vi "TrajectoryGenerate_Make_Cubic_CtrlVect.vi"(8 "traj_config":T7={"MaxVelocity"=0.0, "Max Acceleration"=0.0, "StartVelocity"=0.0, "End Velocity"=0.0, "Reversed"=FALSE, "DiffDrKineConstntDefined"=FALSE, "CentAcellConstntDefined"=FALSE, "DiffDrVoltConstntDefined"=FALSE, "DIFF_DRIVE_KINE_CONSTRAINT"={"Max Speed (M/S)"=0.0, "DIFF_DRIVE_KINEMATICS"={"TrackWidth_Meters"=0.0}}, "CENTRIPETAL_ACCEL_CONSTRAINT"={"Max Cent Accel"=0.0}, "SwerveDrKineConstntDefined"=FALSE, "SWERVE_DRIVE_KINE_CONSTRAINT"={"Max Speed (M/S)"=0.0, "SwerveKinematics"={"NumModules"=0, "InverseKinematics"=[], "ForwardKinematics"=[], "Modules"=[], "PrevCoR"={"X"=0.0, "Y"=0.0}}}, "DIFF_DRIVE_VOLTAGE_CONSTRAINT"={"Max Voltage"=0.0, "DIFF_DRIVE_KINEMATICS"={"TrackWidth_Meters"=0.0}, "SIMPLE_MOTOR_FF"={"Ks"=0.0, "Kv"=0.0, "Ka"=0.0}}, "MECANUM_DRIVE_KINE_CONSTRAINT"={"Max Speed (M/S)"=0.0, "MECA_DRIVE_KINEMATICS"={"FrontLeft"={"X"=0.0, "Y"=0.0}, "FrontRight"={"X"=0.0, "Y"=0.0}, "RearLeft"={"X"=0.0, "Y"=0.0}, "RearRight"={"X"=0.0, "Y"=0.0}, "InverseKinematics"=[[0.0, 1.0, -1.0, 0.0], [0.0, 1.0, 1.0, 0.0], [0.0, 1.0, 1.0, 0.0], [0.0, 1.0, -1.0, 0.0]], "ForwardKinematics"=[[0.0, 1.0, -1.0, 0.0], [0.0, 1.0, 1.0, 0.0], [0.0, 1.0, 1.0, 0.0], [0.0, 1.0, -1.0, 0.0]], "PrevCoR"={"X"=0.0, "Y"=0.0}}}, "MecanumDrKineConstntDefined"=FALSE} {"MECANUM_DRIVE_KINE_CONSTRAINT"."MECA_DRIVE_KINEMATICS"."PrevCoR"."Y" format="%14.3f"; "MECANUM_DRIVE_KINE_CONSTRAINT"."MECA_DRIVE_KINEMATICS"."PrevCoR"."X" format="%14.3f"; "MECANUM_DRIVE_KINE_CONSTRAINT"."MECA_DRIVE_KINEMATICS"."RearRight"."Y" format="%14.3f"; "MECANUM_DRIVE_KINE_CONSTRAINT"."MECA_DRIVE_KINEMATICS"."RearRight"."X" format="%14.3f"; "MECANUM_DRIVE_KINE_CONSTRAINT"."MECA_DRIVE_KINEMATICS"."RearLeft"."Y" format="%14.3f"; "MECANUM_DRIVE_KINE_CONSTRAINT"."MECA_DRIVE_KINEMATICS"."RearLeft"."X" format="%14.3f"; "MECANUM_DRIVE_KINE_CONSTRAINT"."MECA_DRIVE_KINEMATICS"."FrontRight"."Y" format="%14.3f"; "MECANUM_DRIVE_KINE_CONSTRAINT"."MECA_DRIVE_KINEMATICS"."FrontRight"."X" format="%14.3f"; "MECANUM_DRIVE_KINE_CONSTRAINT"."MECA_DRIVE_KINEMATICS"."FrontLeft"."Y" format="%14.3f"; "MECANUM_DRIVE_KINE_CONSTRAINT"."MECA_DRIVE_KINEMATICS"."FrontLeft"."X" format="%14.3f"; "MECANUM_DRIVE_KINE_CONSTRAINT"."Max Speed (M/S)" format="%20.4f"; "DIFF_DRIVE_VOLTAGE_CONSTRAINT"."SIMPLE_MOTOR_FF"."Ka" format="%13.4f"; "DIFF_DRIVE_VOLTAGE_CONSTRAINT"."SIMPLE_MOTOR_FF"."Kv" format="%13.4f"; "DIFF_DRIVE_VOLTAGE_CONSTRAINT"."SIMPLE_MOTOR_FF"."Ks" format="%13.4f"; "DIFF_DRIVE_VOLTAGE_CONSTRAINT"."DIFF_DRIVE_KINEMATICS"."TrackWidth_Meters" format="%20.4f"; "DIFF_DRIVE_VOLTAGE_CONSTRAINT"."Max Voltage" format="%20.4f"; "SWERVE_DRIVE_KINE_CONSTRAINT"."SwerveKinematics"."PrevCoR"."Y" format="%14.3f"; "SWERVE_DRIVE_KINE_CONSTRAINT"."SwerveKinematics"."PrevCoR"."X" format="%14.3f"; "SWERVE_DRIVE_KINE_CONSTRAINT"."SwerveKinematics"."Modules"."Y" format="%14.3f"; "SWERVE_DRIVE_KINE_CONSTRAINT"."SwerveKinematics"."Modules"."X" format="%14.3f"; "SWERVE_DRIVE_KINE_CONSTRAINT"."Max Speed (M/S)" format="%20.4f"; "CENTRIPETAL_ACCEL_CONSTRAINT"."Max Cent Accel" format="%20.4f"; "DIFF_DRIVE_KINE_CONSTRAINT"."DIFF_DRIVE_KINEMATICS"."TrackWidth_Meters" format="%20.4f"; "DIFF_DRIVE_KINE_CONSTRAINT"."Max Speed (M/S)" format="%20.4f"; "End Velocity" format="%20.4f"; "StartVelocity" format="%20.4f"; "Max Acceleration" format="%20.4f"; "MaxVelocity" format="%20.4f"}, 9 "end-Spline_Ctrl_Vector":T1, 10 "Interior WAYPOINTS":T5[](array[typedef]) {"Y" format="%14.3f"; "X" format="%14.3f"}, 11 "initial-Spline_Ctrl_Vector":T1) -> (0 "error out":errorcluster, 3 "TRAJECTORY":T2 {"TotalTImeSecs" format="%20.3f"})   [LabVIEW 2019, in "Trajectory_Library.lvlib"]
doc: "Generates a trajectory from the given control vectors and config. This method uses clamped cubic splines -- a method in which the exterior control vectors and interior waypoints are provided. The headings are automatically determined at the interior points to ensure continuous curvature.\n \nParameters:\n - initialCtrlVector - The initial control vector.\n - interiorWaypoints - The interior waypoints.\n - endCtrlVector - The ending control vector.\n - Trajectory Config - The configuration for the trajectory.\n\nReturns:\n - Trajectory -- Created trajectory data structure\n - Error Out - Returned error cluster"
uses:
  Trajectory_Library.lvlib
  TRANSLATION2D.ctl
  TRAJ_CONFIG.ctl
  TRAJ_CONSTRAINT_DIIF_DRIVE_KINEMATICS.ctl
  DIFF_DRIVE_KINEMATICS.ctl
  TRAJ_CONSTRAINT_CENTRIPETAL_ACCEL.ctl
  TRAJ_CONSTRAINT_SWERVE_DRIVE_KINEMATICS.ctl
  SWERVE_DRIVE_KINEMATICS.ctl
  <vilib>/Analysis/Matrix/Datatypes/RealMatrix.ctl
  TRAJ_CONSTRAINT_DIIF_DRIVE_VOLTAGE.ctl
  SIMPLE_MOTOR_FF.ctl
  TRAJ_CONSTRAINT_MECA_DRIVE_KINEMATICS.ctl
  MECA_DRIVE_KINEMATICS.ctl
  TRAJECTORY.ctl
  TRAJ_STATE.ctl
  POSE2D.ctl
  ROTATION2D.ctl
  SPLINE_CTRL_VECTOR.ctl
  POSEwCURVATURE.ctl
  Pose_TransformBy.vi
  Translation_RotateBy.vi
  Translation_Plus.vi
  Rotation_Plus.vi
  Pose_New_TRRO.vi
  Rotation_RotateBy.vi
  Rotation_CreateXY.vi
  Util_CalcDist.vi
  <vilib>/Analysis/Matrix/NI_Matrix.lvlib
panel:
  # "ARRAY OF OTHER\nCONSTRAINTS \nGOES HERE.."
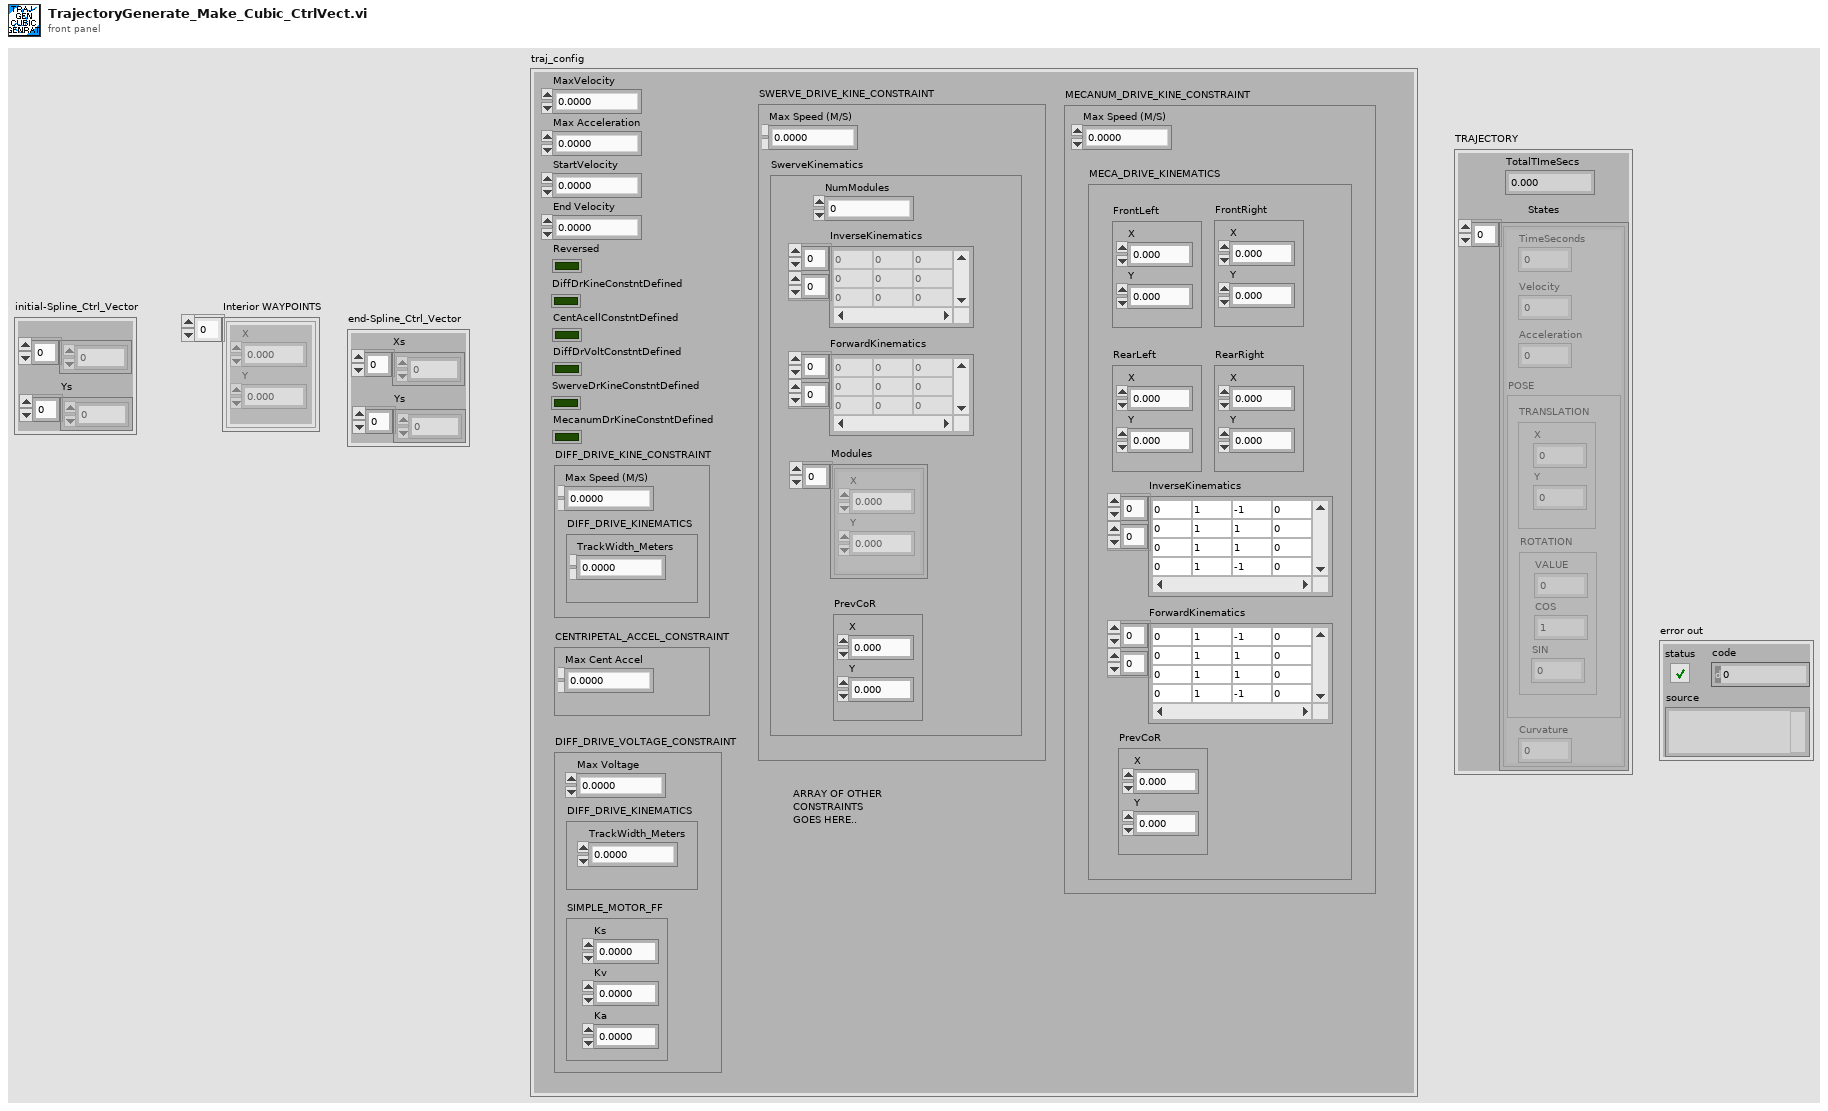
[diagram p1: front panel]
types:
  T1 = typedef "Trajectory_Library.lvlib/SPLINE_CTRL_VECTOR.ctl" = cluster{"Xs":dbl[], "Ys":dbl[]}
  T2 = typedef "Trajectory_Library.lvlib/TRAJECTORY.ctl" = cluster{"TotalTImeSecs":dbl, "States":T3[]}
  T3 = typedef "Trajectory_Library.lvlib/TRAJ_STATE.ctl" = cluster{"TimeSeconds":dbl, "Velocity":dbl, "Acceleration":dbl, "POSE":T4, "Curvature":dbl}
  T4 = typedef "Trajectory_Library.lvlib/POSE2D.ctl" = cluster{"TRANSLATION":T5, "ROTATION":T6}
  T5 = typedef "Trajectory_Library.lvlib/TRANSLATION2D.ctl" = cluster{"X":dbl, "Y":dbl}
  T6 = typedef "Trajectory_Library.lvlib/ROTATION2D.ctl" = cluster{"VALUE":dbl, "COS":dbl, "SIN":dbl}
  T7 = typedef "Trajectory_Library.lvlib/TRAJ_CONFIG.ctl" = cluster{"MaxVelocity":dbl, "Max Acceleration":dbl, "StartVelocity":dbl, "End Velocity":dbl, "Reversed":bool, "DiffDrKineConstntDefined":bool, "CentAcellConstntDefined":bool, "DiffDrVoltConstntDefined":bool, "DIFF_DRIVE_KINE_CONSTRAINT":T8, "CENTRIPETAL_ACCEL_CONSTRAINT":T10, "SwerveDrKineConstntDefined":bool, "SWERVE_DRIVE_KINE_CONSTRAINT":T11, "DIFF_DRIVE_VOLTAGE_CONSTRAINT":T14, "MECANUM_DRIVE_KINE_CONSTRAINT":T16, "MecanumDrKineConstntDefined":bool}
  T8 = typedef "Trajectory_Library.lvlib/TRAJ_CONSTRAINT_DIIF_DRIVE_KINEMATICS.ctl" = cluster{"Max Speed (M/S)":dbl, "DIFF_DRIVE_KINEMATICS":T9}
  T9 = typedef "Trajectory_Library.lvlib/DIFF_DRIVE_KINEMATICS.ctl" = cluster{"TrackWidth_Meters":dbl}
  T10 = typedef "Trajectory_Library.lvlib/TRAJ_CONSTRAINT_CENTRIPETAL_ACCEL.ctl" = cluster{"Max Cent Accel":dbl}
  T11 = typedef "Trajectory_Library.lvlib/TRAJ_CONSTRAINT_SWERVE_DRIVE_KINEMATICS.ctl" = cluster{"Max Speed (M/S)":dbl, "SwerveKinematics":T12}
  T12 = typedef "Trajectory_Library.lvlib/SWERVE_DRIVE_KINEMATICS.ctl" = cluster{"NumModules":i32, "InverseKinematics":T13, "ForwardKinematics":T13, "Modules":T5[], "PrevCoR":T5}
  T13 = typedef "NI_Matrix.lvlib/RealMatrix.ctl" = dbl[][]
  T14 = typedef "Trajectory_Library.lvlib/TRAJ_CONSTRAINT_DIIF_DRIVE_VOLTAGE.ctl" = cluster{"Max Voltage":dbl, "DIFF_DRIVE_KINEMATICS":T9, "SIMPLE_MOTOR_FF":T15}
  T15 = typedef "Trajectory_Library.lvlib/SIMPLE_MOTOR_FF.ctl" = cluster{"Ks":dbl, "Kv":dbl, "Ka":dbl}
  T16 = typedef "Trajectory_Library.lvlib/TRAJ_CONSTRAINT_MECA_DRIVE_KINEMATICS.ctl" = cluster{"Max Speed (M/S)":dbl, "MECA_DRIVE_KINEMATICS":T17}
  T17 = typedef "Trajectory_Library.lvlib/MECA_DRIVE_KINEMATICS.ctl" = cluster{"FrontLeft":T5, "FrontRight":T5, "RearLeft":T5, "RearRight":T5, "InverseKinematics":T13, "ForwardKinematics":T13, "PrevCoR":T5}
  T18 = typedef "Trajectory_Library.lvlib/SPLINE.ctl" = cluster{"Degree":i32, "Coefficients":T13}
  T19 = typedef "Trajectory_Library.lvlib/POSEwCURVATURE.ctl" = cluster{"CURVATURE":dbl, "POSE":T4}
  T20 = typedef "Trajectory_Library.lvlib/TRANSFORM2D.ctl" = cluster{"TRANSLATION":T5, "ROTATION":T6}
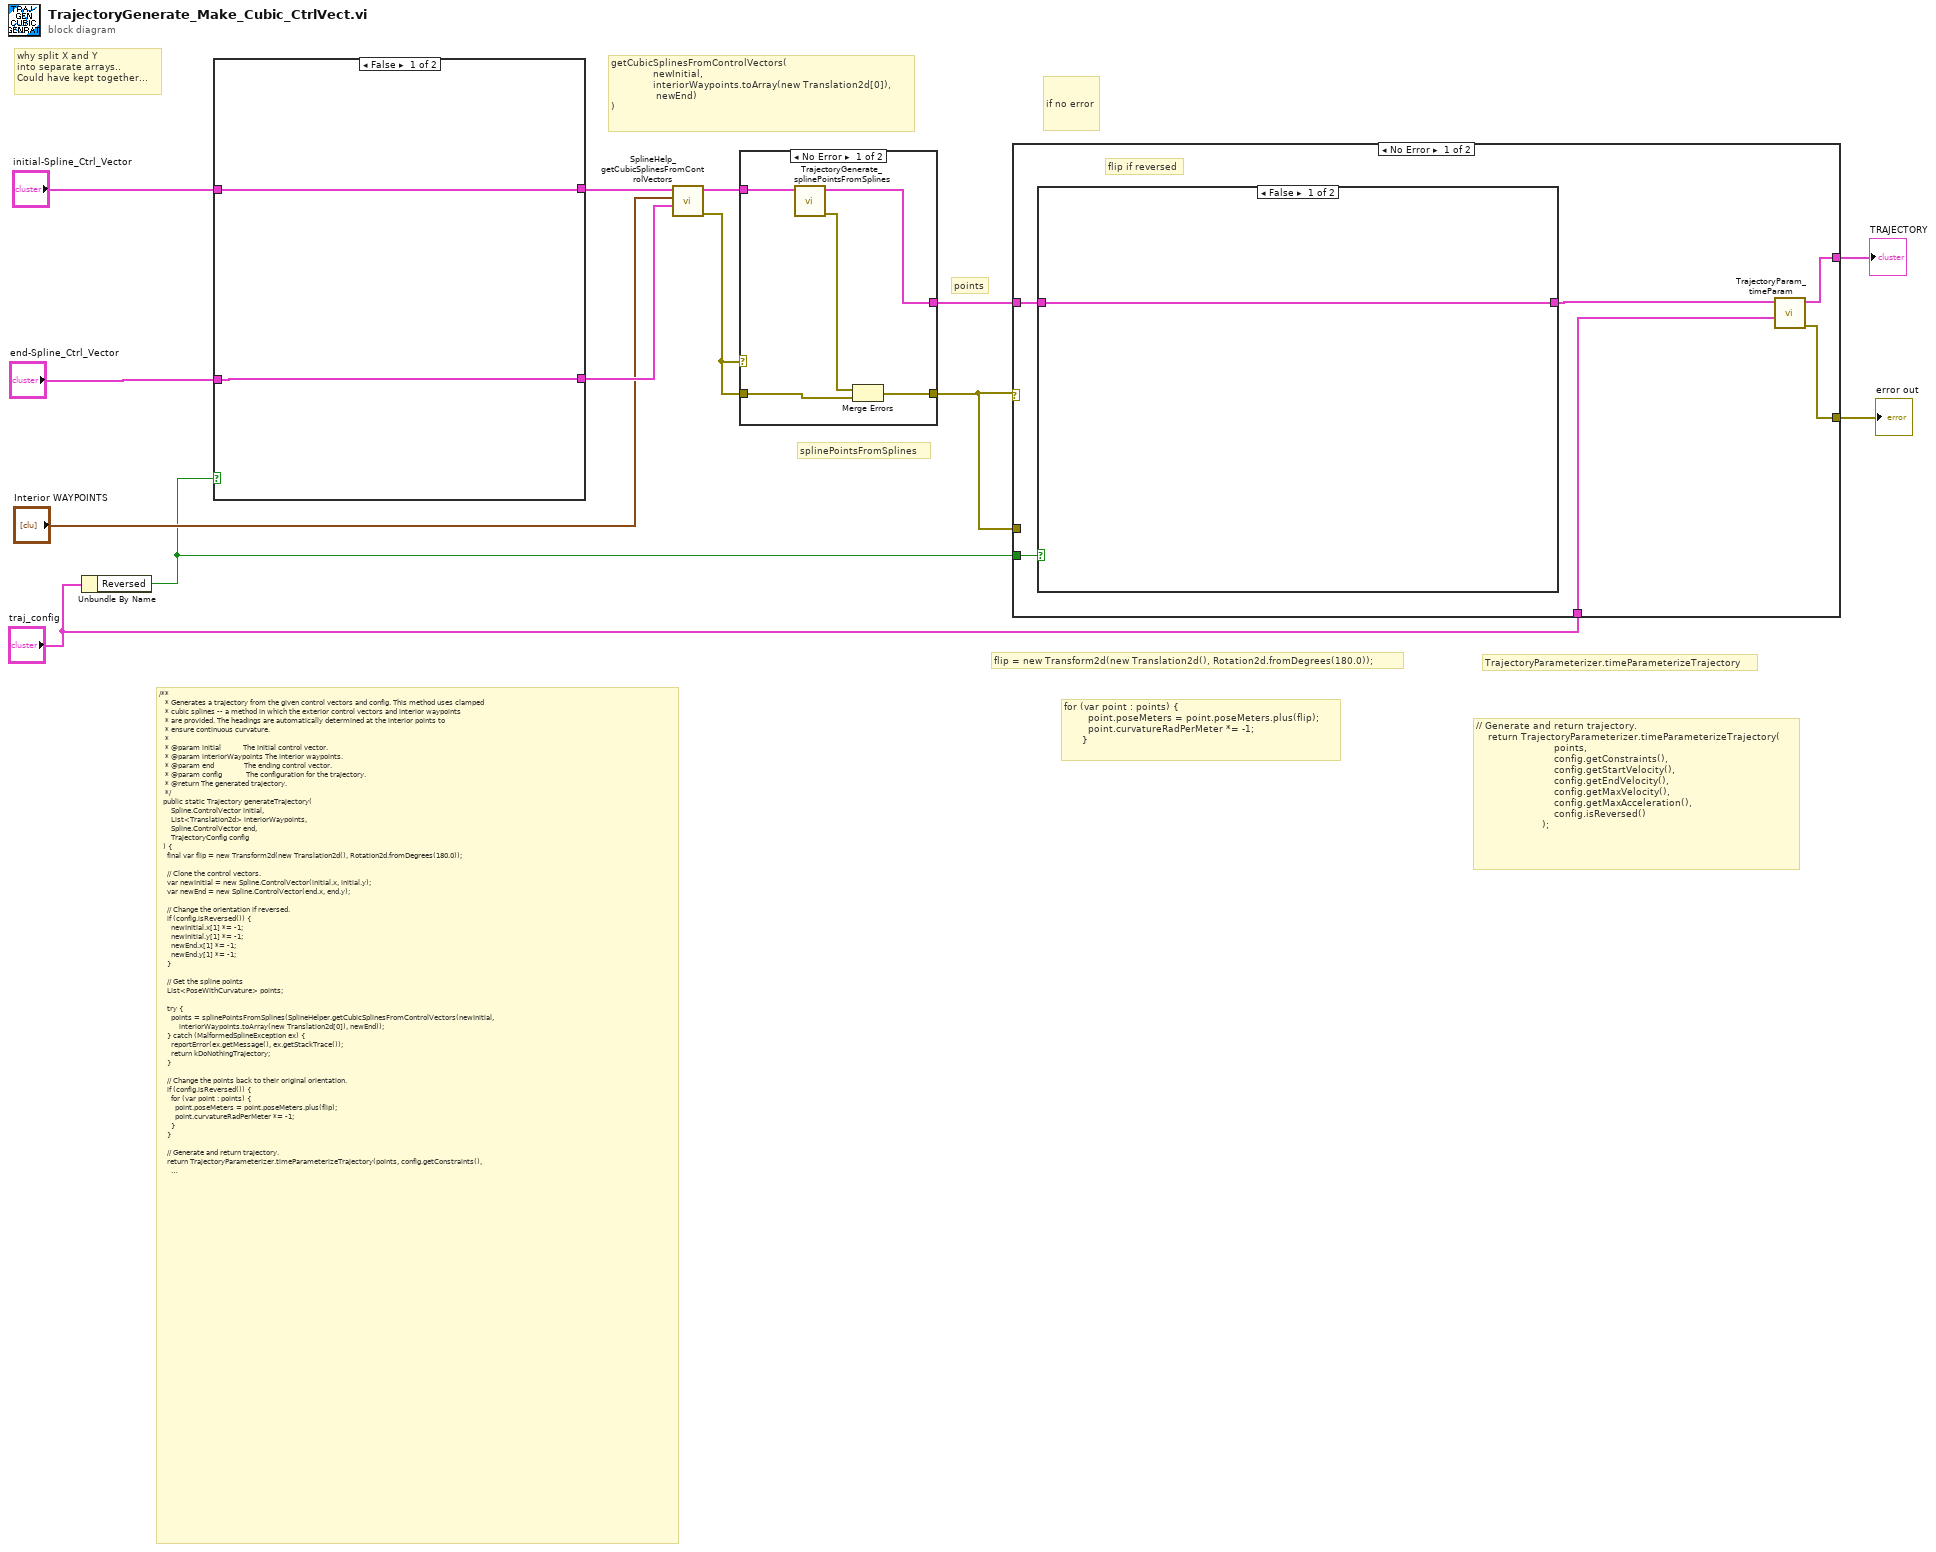
[diagram p0: block diagram]
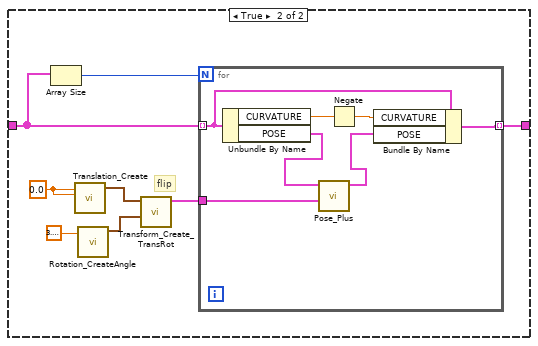
[diagram p2: hidden frame]
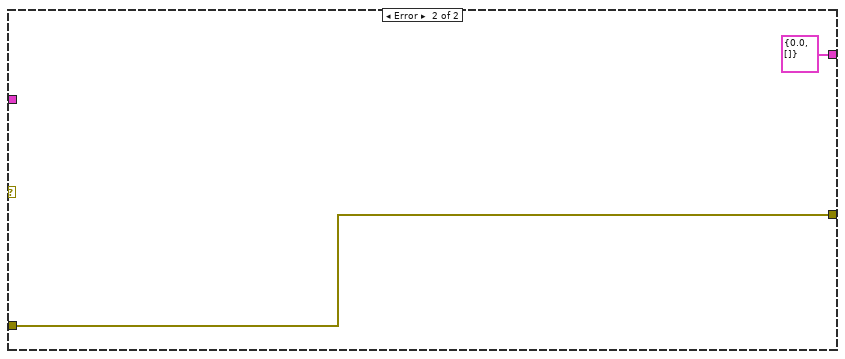
[diagram p3: hidden frame]
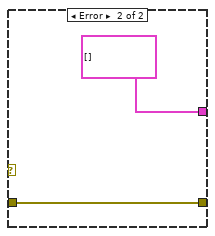
[diagram p4: hidden frame]
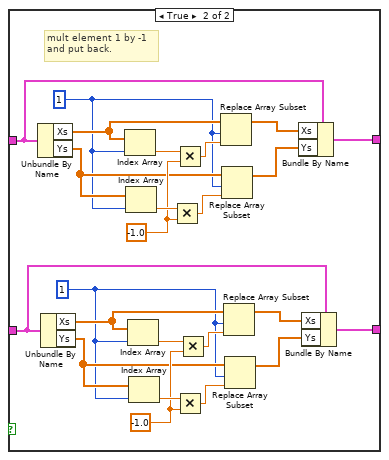
[diagram p5: hidden frame]
diagram:
  # "// Generate and return trajectory.\n    return TrajectoryParameterizer.timeParameterizeTrajectory(\n                          points, \n                          config.getConstraints(),\n                          config.getStartVelocity(), \n                          config.getEndVelocity(), \n                          config.getMaxVelocity(),\n                          config.getMaxAcceleration(), \n                          config.isReversed()\n                      );"
  # "flip = new Transform2d(new Translation2d(), Rotation2d.fromDegrees(180.0));"
  # "for (var point : points) {\n        point.poseMeters = point.poseMeters.plus(flip);\n        point.curvatureRadPerMeter *= -1;\n      }"
  # "points"
  # "TrajectoryParameterizer.timeParameterizeTrajectory"
  # "if no error"
  # "splinePointsFromSplines"
  # "getCubicSplinesFromControlVectors(\n              newInitial,\n              interiorWaypoints.toArray(new Translation2d[0]), \n               newEnd)\n)"
  # "why split X and Y \ninto separate arrays..\nCould have kept together..."
  # "/**\n   * Generates a trajectory from the given control vectors and config. This method uses clamped\n   * cubic splines -- a method in which the exterior control vectors and interior waypoints\n   * are provided. The headings are automatically determined at the interior points to\n   * ensure continuous curvature.\n   *\n   * @param initial           The initial control vector.\n   * @param interiorWaypoints The interior waypoints.\n   * @param end               The ending control vector.\n   * @param config            The configuration for the trajectory.\n   * @return The generated trajectory.\n   */\n  public static Trajectory generateTrajectory(\n      Spline.ControlVector initial,\n      List<Translation2d> interiorWaypoints,\n      Spline.ControlVector end,\n      TrajectoryConfig config\n  ) {\n    final var flip = new Transform2d(new Translation2d(), Rotation2d.fromDegrees(180.0));\n\n    // Clone the control vectors.\n    var newInitial = new Spline.ControlVector(initial.x, initial.y);\n    var newEnd = new Spline.ControlVector(end.x, end.y);\n\n    // Change the orientation if reversed.\n    if (config.isReversed()) {\n      newInitial.x[1] *= -1;\n      newInitial.y[1] *= -1;\n      newEnd.x[1] *= -1;\n      newEnd.y[1] *= -1;\n    }\n\n    // Get the spline points\n    List<PoseWithCurvature> points;\n\n    try {\n      points = splinePointsFromSplines(SplineHelper.getCubicSplinesFromControlVectors(newInitial,\n          interiorWaypoints.toArray(new Translation2d[0]), newEnd));\n    } catch (MalformedSplineException ex) {\n      reportError(ex.getMessage(), ex.getStackTrace());\n      return kDoNothingTrajectory;\n    }\n\n    // Change the points back to their original orientation.\n    if (config.isReversed()) {\n      for (var point : points) {\n        point.poseMeters = point.poseMeters.plus(flip);\n        point.curvatureRadPerMeter *= -1;\n      }\n    }\n\n    // Generate and return trajectory.\n    return TrajectoryParameterizer.timeParameterizeTrajectory(points, config.getConstraints(),\n        config.getStartVelocity(), config.getEndVelocity(), config.getMaxVelocity(),\n        config.getMaxAcceleration(), config.isReversed());\n  }"
  n1 = Unbundle By Name("traj_config") -> ("Reversed"=w6:bool)
  n2 = case shown="False" w6 {
    tunnel: "end-Spline_Ctrl_Vector" -> [w14 w17]
    tunnel: "initial-Spline_Ctrl_Vector" -> [w15 w31]
    tunnel: [w15 w28] -> w11
    tunnel: [w14 w16] -> w10
    frame False {
    }
    frame True {
      w26 = -1.0
      w21 = 1 ("index")
      w38 = -1.0
      w33 = 1 ("index")
      # "mult element 1 by -1\nand put back."
      n3 = Unbundle By Name(w31) -> ("Xs"=w36:dbl[], "Ys"=w34:dbl[])
      n4 = Unbundle By Name(w17) -> ("Xs"=w24:dbl[], "Ys"=w22:dbl[])
      n5 = Index Array(array=w36, index=w33) -> (element=w37:dbl)
      n6 = Index Array(array=w34, index=w33) -> (element=w39:dbl)
      n7 = Index Array(array=w24, index=w21) -> (element=w25:dbl)
      n8 = Index Array(array=w22, index=w21) -> (element=w27:dbl)
      n9 = Multiply(x=w39, y=w38) -> (x*y=w32:dbl)
      n10 = Multiply(x=w37, y=w38) -> (x*y=w35:dbl)
      n11 = Multiply(x=w27, y=w26) -> (x*y=w20:dbl)
      n12 = Multiply(x=w25, y=w26) -> (x*y=w23:dbl)
      n13 = Replace Array Subset(array=w36, new element=w35, index=w33) -> (w30:dbl[])
      n14 = Replace Array Subset(array=w34, new element=w32, index=w33) -> (w29:dbl[])
      n15 = Replace Array Subset(array=w24, new element=w23, index=w21) -> (w19:dbl[])
      n16 = Replace Array Subset(array=w22, new element=w20, index=w21) -> (w18:dbl[])
      n17 = Bundle By Name(cluster=w31, "Xs"=w30, "Ys"=w29) -> (w28:T1)
      n18 = Bundle By Name(cluster=w17, "Xs"=w19, "Ys"=w18) -> (w16:T1)
    }
  }
  n19 = call "SplineHelp_getCubicSplinesFromControlVectors.vi"("endCtrlVector"=w10, "InternalWaypoints"="Interior WAYPOINTS", "startCtrlVector"=w11) -> ("error out"=w8:errorcluster, "splines"=w4:T18[])  [unwired: 3 in, 4 out]
  n20 = case shown="No Error" w8 {
    tunnel: [w44 w46] -> w5
    tunnel: w8 -> [w43 w46]
    tunnel: w4 -> [w41 _]
    tunnel: [w42 T19[] [] ("ArrayPoseWithCurvature")] -> w3
    frame No Error {
      n21 = call "TrajectoryGenerate_splinePointsFromSplines.vi"("inputSPLINE"=w41) -> ("error out"=w40:errorcluster, "ArrayPoseWithCurvature"=w42:T19[])  [unwired: 9 in]
      n22 = Merge Errors(w40, w43) -> (w44:errorcluster)
    }
    frame Error {
    }
  }
  n23 = case shown="No Error" w5 {
    tunnel: w5 -> [_ w70]
    tunnel: [w48 w70] -> w7
    tunnel: w6 -> [w52 _]
    tunnel: w3 -> [w51 _]
    tunnel: [w49 T2 {"TotalTImeSecs"=0.0, "States"=[]} ("TRAJECTORY")] -> w2
    tunnel: "traj_config" -> [w47 _]
    frame No Error {
      # "flip if reversed"
      n24 = case shown="False" w52 {
        tunnel: w51 -> [w53 w60]
        tunnel: [w53 w59] -> w50
        frame False {
        }
        frame True {
          w55 = 0.0 ("X")
          # "flip"
          n25 = Array Size(array=w60) -> (size(s)=w61:i32)
          n26 = call "Translation_Create.vi"("Y"=w55, "X"=w55) -> ("TRANSLATION"=w57:T5)  [unwired: 9 in]
          n27 = call "Rotation_CreateAngle.vi"("Angle"=3.141592653589793) -> ("ROTATION"=w58:T6)  [unwired: 10 in]
          n28 = call "Transform_Create_TransRot.vi"("ROTATION"=w58, "TRANSLATION"=w57) -> ("TRANSFORM"=w54:T20)  [unwired: 9 in]
          n29 = for {
            N: w61 -> [_]
            tunnel: w60 -> [w67] mode=indexing
            tunnel: [w66] -> w59 mode=indexing
            tunnel: w54 -> [w64]
            n30 = Unbundle By Name(w67) -> ("CURVATURE"=w68:dbl, "POSE"=w63:T4)
            n31 = call "Pose_Plus.vi"("other TRANSFORM"=w64, "in POSE"=w63) -> ("out POSE"=w62:T4)  [unwired: 9 in]
            n32 = Negate(x=w68) -> (-x=w65:dbl)
            n33 = Bundle By Name(cluster=w67, "CURVATURE"=w65, "POSE"=w62) -> (w66:T19)
          }
        }
      }
      n34 = call "TrajectoryParam_timeParam.vi"("TRAJECTORY_CONFIG"=w47, "points"=w50) -> ("error out"=w48:errorcluster, "TRAJECTORY"=w49:T2)  [unwired: 8 in]
    }
    frame Error {
    }
  }
  "TRAJECTORY" <- w2
  "error out" <- w7
